vi "GT Get Adc.vi"(6 "pClock":u32, 7 "count":i16, 8 "error in (no error)":errorcluster caption="错误输入（无错误）", 9 "pValue":dbl[](array[numeric]), 10 "adc":i16, 11 "cardNum":i16) -> (0 "error out":errorcluster caption="错误输出", 1 "pValue out":dbl[](array[numeric]), 3 "function return":i16, 4 "pClock out":u32)   [LabVIEW 2014, in "gts.lvlib"]
doc: "GT_API GT_GetAdc(short cardNum,short adc,double *pValue,short count=1,unsigned long *pClock=NULL);"
uses:
  gts.lvlib
  gts.dll
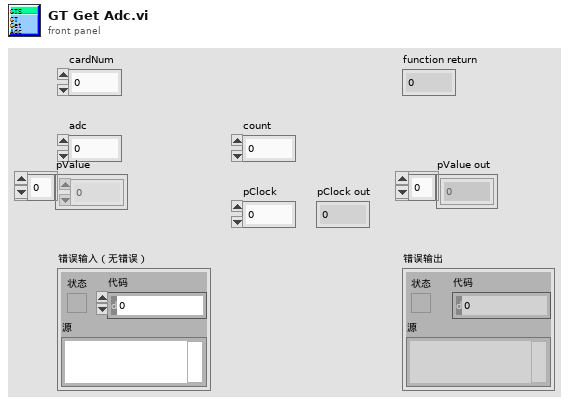
[diagram p1: front panel]
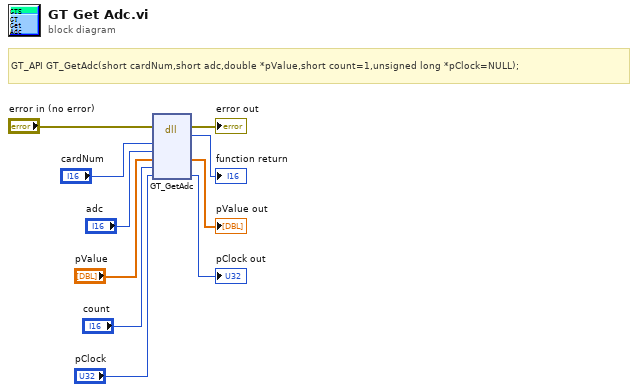
[diagram p0: block diagram]
diagram:
  # "GT_API GT_GetAdc(short cardNum,short adc,double *pValue,short count=1,unsigned long *pClock=NULL);"
  n1 = dll-call lib="PTH2kabs D固高科技资料LABVIEWlabview 例程.多卡库-控制卡基本运动例程(labview)gts.*" fn="GT_GetAdc"(error in="error in (no error)", "cardNum"="cardNum", "adc"="adc", "pValue"="pValue", "count"="count", "pClock"="pClock") -> (error out=→"error out":errorcluster, "返回类型"=→"function return":i16, "pValue"=→"pValue out":dbl[], "pClock"=→"pClock out":u32)  [unwired: 5 in, 1 out]
